vi "StatusGood.vi"(10 "Text.Text":string, 11 "String in":refnum<vi>) -> ()   [LabVIEW 2020]
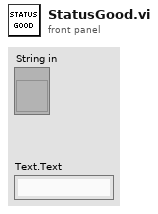
[diagram p1: front panel]
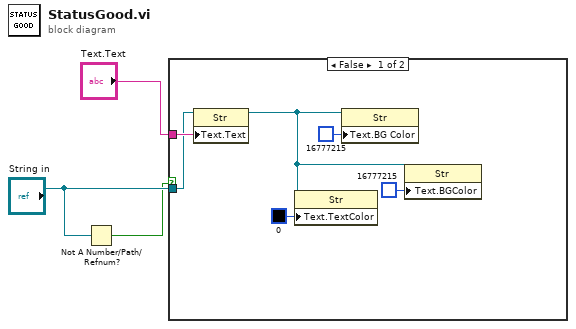
[diagram p0: block diagram]
diagram:
  n1 = Not A Number/Path/Refnum?(number/path/refnum="String in") -> (NaN/Path/Refnum?=w1:bool)
  n2 = case shown="False" w1 {
    tunnel: "Text.Text" -> [w5 _]
    tunnel: "String in" -> [w4 _]
    frame False {
      n3 = property class="Str"(reference=w4, "Text.Text"=w5) -> (reference out=w8:refnum<vi>)  [unwired: 1 in, 1 out]
      n4 = property class="Str"(reference=w8, "Text.TextColor"=u32 0 ("Text.Text Colors:Text Color")) -> ()  [unwired: 1 in, 2 out]
      n5 = property class="Str"(reference=w8, "Text.BG Color"=u32 16777215 ("Text.Colors:BG Color")) -> ()  [unwired: 1 in, 2 out]
      n6 = property class="Str"(reference=w8, "Text.BGColor"=u32 16777215 ("Text.Text Colors:BG Color")) -> ()  [unwired: 1 in, 2 out]
    }
    frame True {
    }
  }
